vi "Fire Display Event.vi"(8 "error in (no error)":errorcluster, 10 "Graph Data":waveform(dbl)[](array[waveform]), 11 "Acquisition UI in":refnum<class "Acquisition UI.lvclass">) -> (0 "error out":errorcluster, 3 "Acquisition UI out":refnum<class "Acquisition UI.lvclass">)   [LabVIEW 2018, in "Acquisition UI.lvlib" / "Acquisition UI.lvclass"]
uses:
  Acquisition UI.lvclass
  Acquisition UI.lvclass/Acquisition UI.ctl
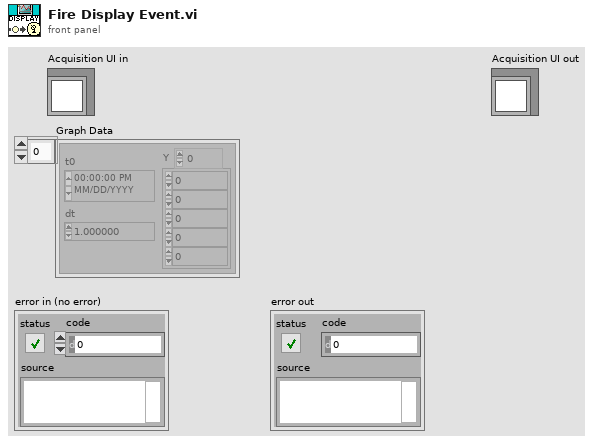
[diagram p1: front panel]
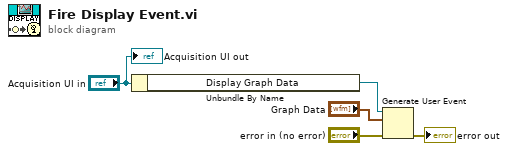
[diagram p0: block diagram]
diagram:
  n1 = Unbundle By Name("Acquisition UI in") -> ("Display Graph Data"=w1:refnum<user-event>)
  n2 = Generate User Event(user event=w1, event data cluster="Graph Data", error in="error in (no error)") -> (error out=→"error out":errorcluster)  [unwired: 1 in, 1 out]
  "Acquisition UI out" <- "Acquisition UI in"
